vi "prepractica 5.vi"() -> ()   [LabVIEW 2015]
panel:
  out "Res. conversión":dbl
  in  "Valor a convertir":dbl
  in  "Seleccione un tipo de conversión":string(combo)
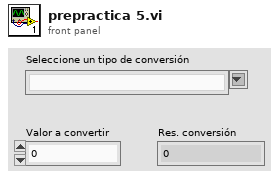
[diagram p1: front panel]
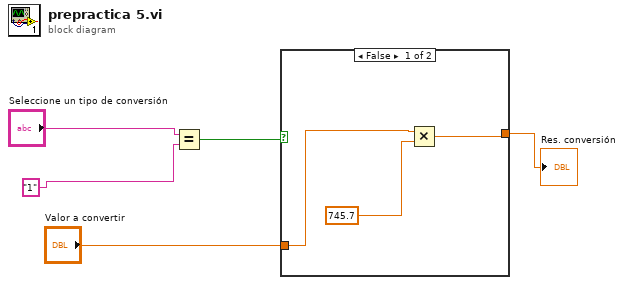
[diagram p0: block diagram]
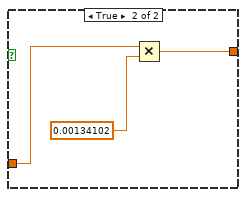
[diagram p2: hidden frame]
diagram:
  n1 = Equal?(x="Seleccione un tipo de conversión", y="1") -> (x = y?=w3:bool)
  n2 = case shown="False" w3 {
    tunnel: "Valor a convertir" -> [w8 w10]
    tunnel: [w6 w9] -> w1
    frame False {
      n3 = Multiply(x=w8, y=745.7 ("Numeric")) -> (x*y=w6:dbl)
    }
    frame True {
      n4 = Multiply(x=w10, y=0.00134102 ("Numeric")) -> (x*y=w9:dbl)
    }
  }
  "Res. conversión" <- w1
